vi "Shuai move.vi"(1 "Color":i32, 2 "Array Position":cluster{"Row":i32, "Column":i32}, 3 "Chess Array":i32[][](array[numeric])=[[140, 130, 120, 110, 100, 111, 121, 131, 141], [-1, -1, -1, -1, -1, -1, -1, -1, -1], [-1, 150, -1, -1, -1, -1, -1, 151, -1], [160, -1, 161, -1, 162, -1, 163, -1, 164], [-1, -1, -1, -1, -1, -1, -1, -1, -1], [-1, -1, -1, -1, -1, -1, -1, -1, -1], [260, -1, 261, -1, 262, -1, 263, -1, 264], [-1, 250, -1, -1, -1, -1, -1, 251, -1], [-1, -1, -1, -1, -1, -1, -1, -1, -1], [240, 230, 220, 210, 200, 211, 221, 231, 241]]) -> (0 "Shuai move":cluster{i32, i32}[](array[cluster]))   [LabVIEW 2009]
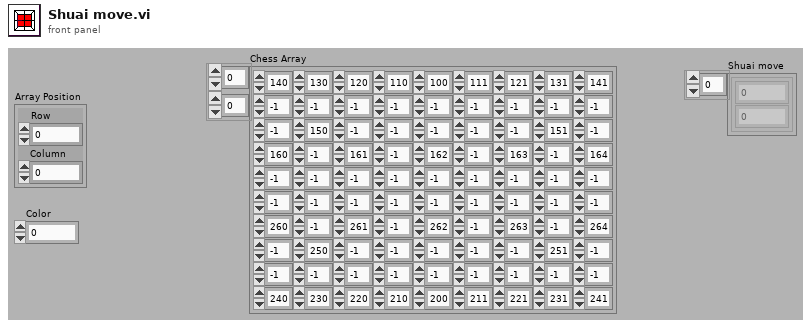
[diagram p1: front panel]
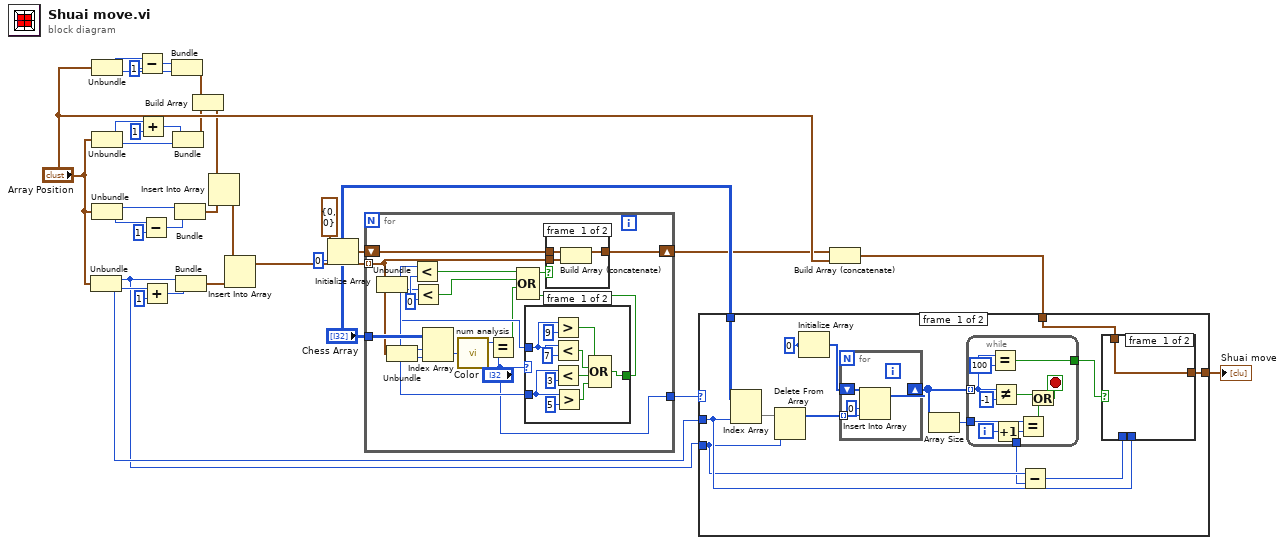
[diagram p0: block diagram]
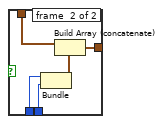
[diagram p2: hidden frame]
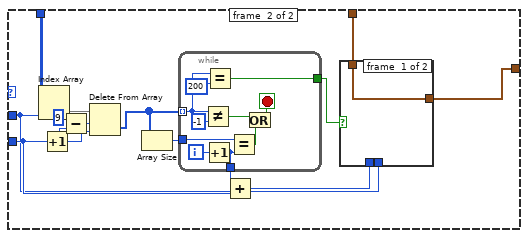
[diagram p3: hidden frame]
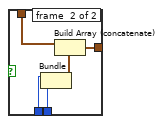
[diagram p4: hidden frame]
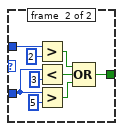
[diagram p5: hidden frame]
diagram:
  n1 = Unbundle("Array Position") -> ("Row"=w4:i32, "Column"=w5:i32)
  n2 = Unbundle("Array Position") -> ("Row"=w6:i32, "Column"=w32:i32)
  n3 = Unbundle("Array Position") -> ("Row"=w31:i32, "Column"=w28:i32)
  n4 = Unbundle("Array Position") -> ("Row"=w27:i32, "Column"=w29:i32)
  n5 = Subtract(x=w6, y=1) -> (x-y=w15:i32)
  n6 = Add(x=w31, y=1) -> (x+y=w13:i32)
  n7 = Subtract(x=w29, y=1) -> (x-y=w11:i32)
  n8 = Add(x=w5, y=1) -> (x+y=w9:i32)
  n9 = Bundle(w15, "Column"=w32) -> (w22:cluster{i32, "Column":i32})  [unwired: 1 out]
  n10 = Bundle(w13, "Column"=w28) -> (w21:cluster{i32, "Column":i32})  [unwired: 1 out]
  n11 = Bundle("Row"=w27, w11) -> (w19:cluster{"Row":i32, i32})  [unwired: 1 out]
  n12 = Bundle("Row"=w4, w9) -> (w17:cluster{"Row":i32, i32})  [unwired: 1 out]
  n13 = Build Array(w22, w21) -> (w20:cluster{i32, "Column":i32}[])
  n14 = Insert Into Array(array=w20, new element=w19) -> (w18:cluster{i32, "Column":i32}[])  [unwired: 1 in]
  n15 = Insert Into Array(array=w18, new element=w17) -> (w26:cluster{i32, "Column":i32}[])  [unwired: 1 in]
  n16 = Initialize Array(cluster{i32, i32} {0, 0} ("Output Cluster"), 0 ("Dimension Size")) -> (w25:cluster{i32, i32}[])
  n17 = for {
    tunnel: w26 -> [w37] mode=indexing
    shift-right: [w44] -> w3
    shift-left: w25 -> [w45]
    tunnel: "Chess Array" -> [w43]
    tunnel: ["Color"] -> w7
    w49 = 0 ("y")
    n18 = Unbundle(w37) -> (w36:i32, "Column"=w40:i32)
    n19 = Unbundle(w37) -> (w39:i32, "Column"=w38:i32)
    n20 = Less?(x=w36, y=w49) -> (x < y?=w47:bool)
    n21 = Less?(x=w40, y=w49) -> (x < y?=w48:bool)
    n22 = Index Array(array=w43, index (row)=w39, index (col)=w38) -> (element=w42:i32)
    n23 = call "num analysis.vi"("x"=w42) -> ("Color"=w41:i32)  [unwired: 2 out]
    n24 = Equal?(x=w41, y="Color") -> (x = y?=w35:bool)
    n25 = case shown="1, Default" "Color" {
      tunnel: w36 -> [w52 w68]
      tunnel: w40 -> [w57 w66]
      tunnel: [w60 w69] -> w34
      frame #0 {
        n26 = Greater?(x=w52, y=9) -> (0:w50:bool)
        n27 = Less?(x=w52, y=7) -> (x < y?=w55:bool)
        n28 = Less?(x=w57, y=3) -> (x < y?=w54:bool)
        n29 = Greater?(x=w57, y=5) -> (0:w53:bool)
        n30 = Compound Arithmetic op=OR(w50, w55, w54, w53) -> (w60:bool)
      }
      frame #1 {
        n31 = Greater?(x=w68, y=2) -> (0:w64:bool)
        n32 = Less?(x=w66, y=3) -> (x < y?=w63:bool)
        n33 = Greater?(x=w66, y=5) -> (0:w62:bool)
        n34 = Compound Arithmetic op=OR(w64, w63, w62) -> (w69:bool)
      }
    }
    n35 = Compound Arithmetic op=OR(w47, w48, w35, w34) -> (w46:bool)
    n36 = case shown="False" w46 {
      tunnel: w45 -> [w72 w73]
      tunnel: [w71 w73] -> w44
      tunnel: w37 -> [w70 _]
      frame #0 {
        n37 = Build Array (concatenate)(w72, w70) -> (w71:cluster{i32, "Column":i32}[])
      }
      frame #1 {
      }
    }
  }
  n38 = Build Array (concatenate)(w3, "Array Position") -> (w1:cluster{"Row":i32, "Column":i32}[])
  n39 = case shown="1, Default" w7 {
    tunnel: w5 -> [w79 w114]
    tunnel: w4 -> [w78 w116]
    tunnel: "Chess Array" -> [w87 w121]
    tunnel: w1 -> [w81 w113]
    tunnel: [w75 w112] -> w2
    frame #0 {
      w85 = 0
      n40 = Index Array(array=w87, index (col)=w79) -> (element=w74:i32[])  [unwired: 1 in]
      n41 = Delete From Array(array=w74, length=w78, index=w78) -> (array with subset deleted=w86:i32[])  [unwired: 1 out]
      n42 = Initialize Array(w85, w85) -> (w84:i32[])
      n43 = for {
        tunnel: w86 -> [w105] mode=indexing
        shift-right: [w104] -> w83
        shift-left: w84 -> [w107]
        n44 = Insert Into Array(array=w107, index=0 ("Index"), new element=w105) -> (w104:i32[])
      }
      n45 = Array Size(array=w83) -> (size(s)=w82:i32)
      n46 = while {
        tunnel: w83 -> [w97] mode=indexing
        tunnel: w82 -> [w99]
        tunnel: [w95] -> w80
        tunnel: [w94] -> w77
        i -> [w102]
        stop <- w100 stop-if-true
        n47 = Equal?(x=w97, y=100) -> (x = y?=w95:bool)
        n48 = Not Equal?(x=w97, y=-1) -> (x != y?=w98:bool)
        n49 = Increment(x=w102) -> (x+1=w94:i32)
        n50 = Equal?(x=w99, y=w94) -> (x = y?=w101:bool)
        n51 = Or(x=w98, y=w101) -> (x .or. y?=w100:bool)
      }
      n52 = Subtract(x=w78, y=w77) -> (x-y=w76:i32)
      n53 = case shown="True" w80 {
        tunnel: w79 -> [_ w92]
        tunnel: w76 -> [_ w93]
        tunnel: w81 -> [w88 w91]
        tunnel: [w88 w89] -> w75
        frame #0 {
        }
        frame #1 {
          n54 = Bundle(w93, "Column"=w92) -> (w90:cluster{i32, "Column":i32})  [unwired: 1 out]
          n55 = Build Array (concatenate)(w91, w90) -> (w89:cluster{"Row":i32, "Column":i32}[])
        }
      }
    }
    frame #1 {
      n56 = Index Array(array=w121, index (col)=w114) -> (element=w111:i32[])  [unwired: 1 in]
      n57 = Increment(x=w116) -> (x+1=w108:i32)
      n58 = Subtract(x=9, y=w116) -> (x-y=w109:i32)
      n59 = Delete From Array(array=w111, length=w109, index=w108) -> (deleted portion=w120:i32[])  [unwired: 1 out]
      n60 = Array Size(array=w120) -> (size(s)=w119:i32)
      n61 = while {
        tunnel: w120 -> [w131] mode=indexing
        tunnel: w119 -> [w132]
        tunnel: [w129] -> w118
        tunnel: [w128] -> w117
        i -> [w136]
        stop <- w133 stop-if-true
        n62 = Not Equal?(x=w131, y=-1) -> (x != y?=w134:bool)
        n63 = Increment(x=w136) -> (x+1=w128:i32)
        n64 = Equal?(x=w131, y=200) -> (x = y?=w129:bool)
        n65 = Equal?(x=w132, y=w128) -> (x = y?=w135:bool)
        n66 = Or(x=w134, y=w135) -> (x .or. y?=w133:bool)
      }
      n67 = Add(x=w117, y=w116) -> (x+y=w115:i32)
      n68 = case shown="True" w118 {
        tunnel: w115 -> [_ w124]
        tunnel: w114 -> [_ w123]
        tunnel: w113 -> [w122 w127]
        tunnel: [w122 w125] -> w112
        frame #0 {
        }
        frame #1 {
          n69 = Bundle(w124, "Column"=w123) -> (w126:cluster{i32, "Column":i32})  [unwired: 1 out]
          n70 = Build Array (concatenate)(w127, w126) -> (w125:cluster{"Row":i32, "Column":i32}[])
        }
      }
    }
  }
  "Shuai move" <- w2
